vi "MF-101 Serial write and read on same channel.vi"() -> ()   [LabVIEW 8.6]
uses:
  <libdir>/resource/objmgr/ueidaq.rc
  vi.lib/UeiDaq/UeiDaqConfigureTimingForSimpleIO.vi
  vi.lib/UeiDaq/UeiDaqCreateSerialSession.vi
  vi.lib/UeiDaq/UeiDaqReadOneDigitalScanUInt16.vi
  vi.lib/UeiDaq/UeiDaqCreateDISession.vi
  vi.lib/UeiDaq/UeiDaqCreateDOSession.vi
  vi.lib/UeiDaq/UeiDaqWriteOneDigitalScanUInt16.vi
  vi.lib/UeiDaq/UeiDaqConfigureTimingForMessagingIO.vi
panel:
  out "DO raw data":u32[](array[numeric]) format="%b"
  out "Total scans":u32
  in  "TRIGOUT":bool
  out "DI TTL Port":bool[][](array[boolean])
  out "Total scans acquired":u32
  in  "Digital Output Resource":string
  in  "Digital Input Resource":string
  out "Available bytes":i32[](array[numeric])
  in  "Append":bool
  in  "Clear":bool
  out "Timeout":bool
  in  "Bits per second":i32(ring) items=["110 bitsPerSecond", "300 bitsPerSecond", "600 bitsPerSecond", "1200 bitsPerSecond", "2400 bitsPerSecond", "4800 bitsPerSecond", "9600 bitsPerSecond", "14400 bitsPerSecond", "19200 bits PerSecond", "28800 bitsPerSecond", "38400 bitsPerSecond", "57600 bitsPerSecond", "115200 bitsPerSecond", "128000 bitsPerSecond", "256000 bitsPerSecond"]
  in  "Stop bits":i32(ring) items=["1 stop bit", "1.5 stop bits", "2 stop bits"]
  in  "Parity":i32(ring) items=["None", "Odd", "Even"]
  in  "Data bits":i32(ring) items=["5 data bits", "6 data bits", "7 data bits", "8 data bits"]
  out "string from serial port":string
  in  "String to send to serial port":string
  in  "Send":bool
  out "return count":i32
  out "device name":string
  in  "Serial Resource":string
  in  "stop":bool
  # "MF-101 Write & Read Serial Port"
  # "1/ Set the resource name -->"
  # "TRUE  = RS232\nFALSE = RS422/485"
  # "2/ Configure Serial port -->"
  # "3/ Send/Receive -->"
  # "Device info"
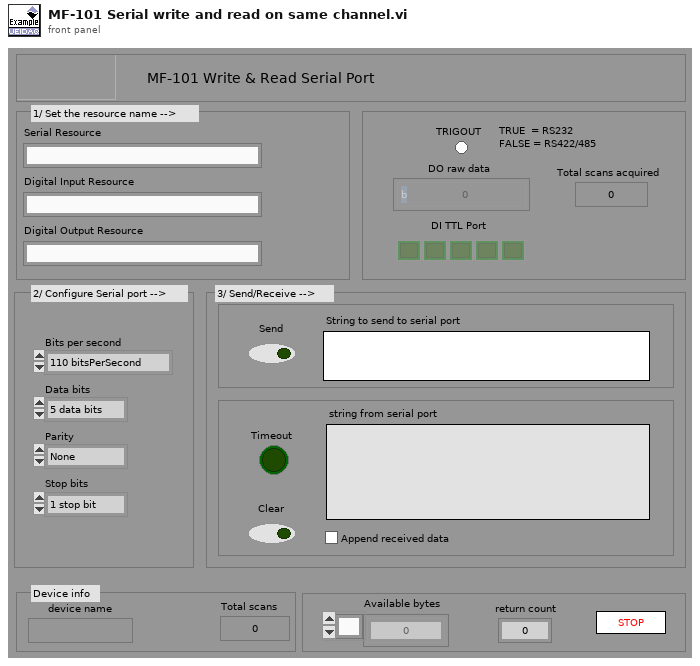
[diagram p1: front panel]
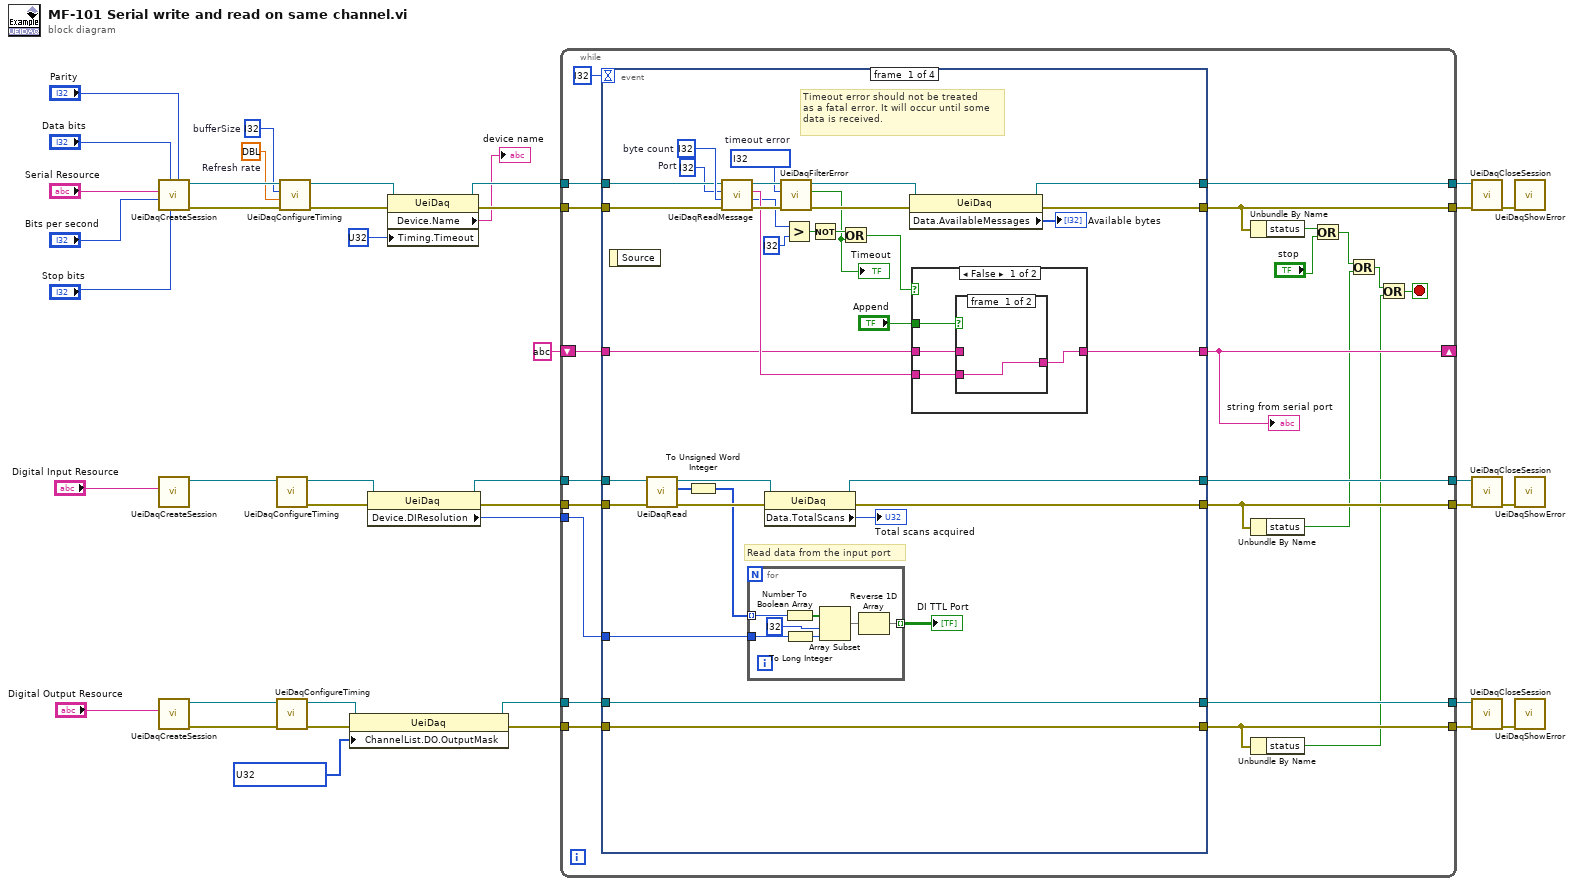
[diagram p0: block diagram]
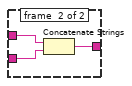
[diagram p2: hidden frame]
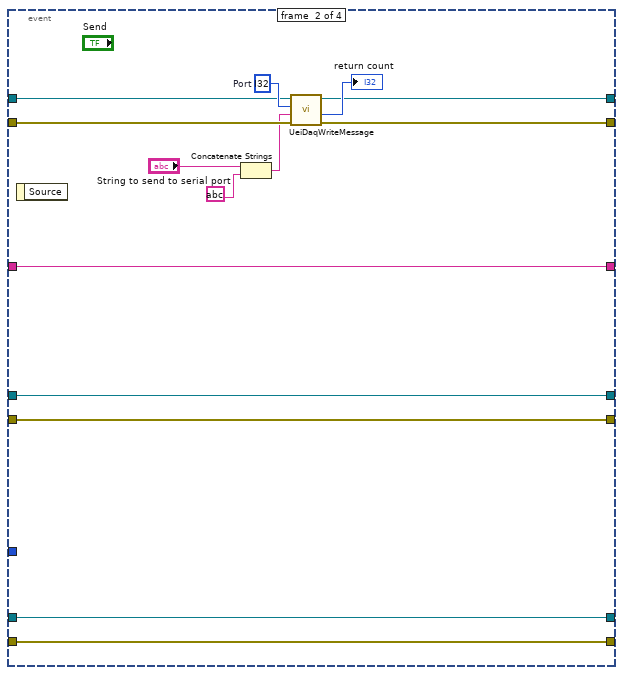
[diagram p4: hidden frame]
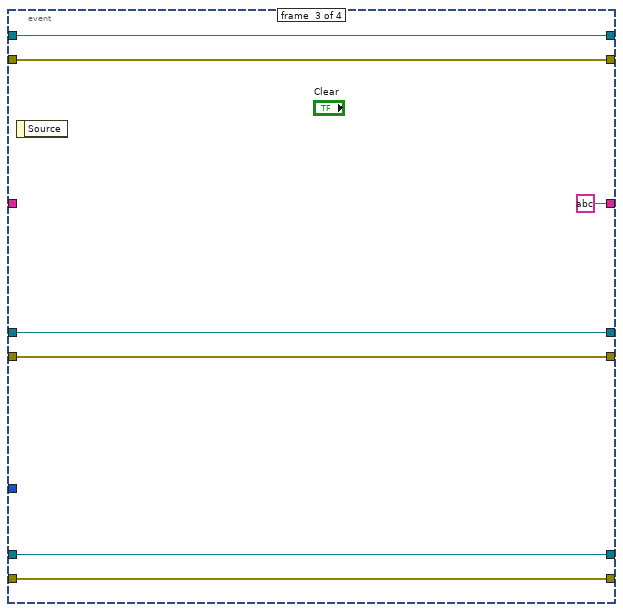
[diagram p5: hidden frame]
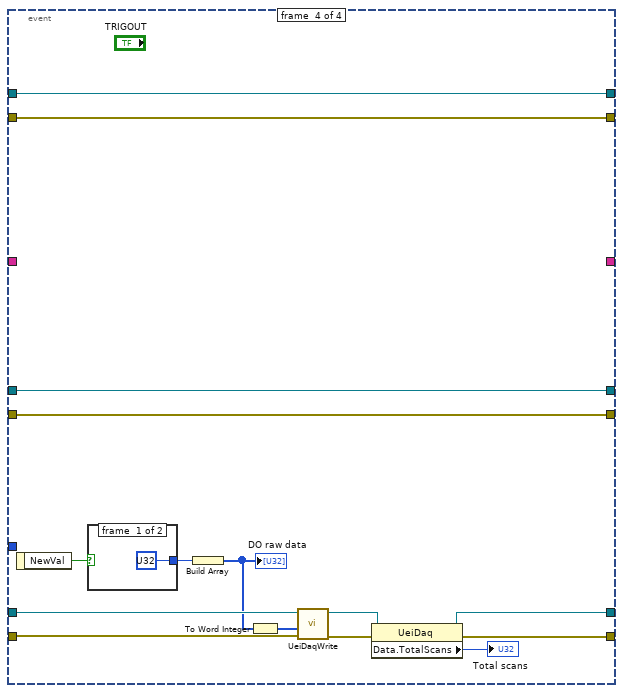
[diagram p6: hidden frame]
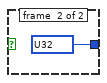
[diagram p7: hidden frame]
diagram:
  w1 = i32 ?  # bufferSize
  w2 = dbl ?  # Refresh rate
  n1 = call-poly "UeiDaqCreateSession.vi"("Parity"="Parity", "Stop bits"="Stop bits", "Data bits"="Data bits", "Bits per second"="Bits per second", "Resource"="Serial Resource") -> ("error out"=w37:errorcluster, "UeiDaq Refnum Out"=w38:refnum<k20>)  [unwired: 4 in, 1 out]
  n2 = call-poly "UeiDaqCreateSession.vi"("Resource"="Digital Input Resource") -> ("UeiDaq Refnum Out"=w8:refnum<k20>)  [unwired: 2 in, 8 out]
  n3 = call-poly "UeiDaqCreateSession.vi"("Resource"="Digital Output Resource") -> ("error out"=w22:errorcluster, "UeiDaq Refnum Out"=w23:refnum<k20>)  [unwired: 3 in, 6 out]
  n4 = call-poly "UeiDaqConfigureTiming.vi"("UeiDaq Refnum In"=w8) -> ("error out"=w6:errorcluster, "UeiDaq Refnum Out"=w7:refnum<k20>)  [unwired: 2 in, 7 out]
  n5 = call-poly "UeiDaqConfigureTiming.vi"("error in (no error)"=w22, "UeiDaq Refnum In"=w23) -> ("error out"=w20:errorcluster, "UeiDaq Refnum Out"=w21:refnum<k20>)  [unwired: 1 in, 7 out]
  n6 = call-poly "UeiDaqConfigureTiming.vi"("error in (no error)"=w37, "Refresh rate"=w2, "bufferSize"=w1, "UeiDaq Refnum In"=w38) -> ("error out"=w33:errorcluster, "UeiDaq Refnum Out"=w35:refnum<k20>)  [unwired: 6 out]
  n7 = property class="UeiDaq"(reference=w21, error in=w20, "ChannelList.DO.OutputMask"=u32[] ? ("Output Mask")) -> (reference out=w11:refnum<k20>, error out=w10:errorcluster)
  n8 = property class="UeiDaq"(reference=w7, error in=w6) -> (reference out=w3:refnum<k20>, error out=w4:errorcluster, "Device.DIResolution"=w5:u32)
  n9 = property class="UeiDaq"(reference=w35, error in=w33, "Timing.Timeout"=u32 ? ("Timing:Timeout")) -> (reference out=w34:refnum<k20>, error out=w32:errorcluster, "Device.Name"=→"device name":string)
  n10 = while {
    tunnel: w34 -> [w62]
    tunnel: w32 -> [w63]
    tunnel: [w59] -> w31
    tunnel: [w60] -> w30
    shift-right: [w56] -> _
    shift-left: string ? ("Message") -> [w57]
    tunnel: w3 -> [w55]
    tunnel: w4 -> [w54]
    tunnel: w11 -> [w50]
    tunnel: w10 -> [w49]
    tunnel: w5 -> [w53]
    tunnel: [w52] -> w16
    tunnel: [w51] -> w15
    tunnel: [w48] -> w13
    tunnel: [w47] -> w12
    stop <- w41 stop-if-true
    n11 = event shown="[3] \"TRIGOUT\": Value Change" {
      selector: _ -> [_ _ _ _]
      dyn-events: _ -> [_ _ _ _]
      timeout: i32 ? -> [_ _ _ _]
      tunnel: w63 -> [w96 w125 w129 w136]
      tunnel: w62 -> [w97 w126 w130 w137]
      tunnel: [w90 w123 _ w137] -> w60
      tunnel: [w88 w124 w129 w136] -> w59
      tunnel: [w86 w119 string ? ("Message") _] -> w56
      tunnel: w57 -> [w85 w119 _ _]
      tunnel: w55 -> [w75 w116 w134 w139]
      tunnel: w54 -> [w76 w115 w133 w138]
      tunnel: [w74 w116 w134 w139] -> w52
      tunnel: w53 -> [w73 _ _ _]
      tunnel: [w72 w115 w133 w138] -> w51
      tunnel: w50 -> [w71 w118 w132 w147]
      tunnel: w49 -> [w70 w117 w131 w146]
      tunnel: [w71 w118 w132 w145] -> w48
      tunnel: [w70 w117 w131 w144] -> w47
      tunnel: [_ _ w130 _] -> _
      event #0 {
        w83 = i32 ?  # Port
        w92 = i32 ?  # timeout error
        w98 = i32 ?  # byte count
        # "Read data from the input port"
        # "Timeout error should not be treated\nas a fatal error. It will occur until some\ndata is received."
        n12 = event-data() -> ()  [unwired: 2 out]
        n13 = call-poly "UeiDaqRead.vi"("error in (no error)"=w76, "UeiDaq Refnum In"=w75) -> ("error out"=w78:errorcluster, "Raw Data"=w81:i16[], "UeiDaq Refnum Out"=w79:refnum<k20>)  [unwired: 7 out]
        n14 = To Unsigned Word Integer(number=w81) -> (unsigned 16bit integer=w77:u16[])
        n15 = call "UeiDaqReadMessage.vi"("error in (no error)"=w96, "byte count"=w98, "Port"=w83, "UeiDaq Refnum In"=w97) -> ("error out"=w94:errorcluster, "return count"=w69:i32, "Message"=w93:string, "UeiDaq Refnum Out"=w95:refnum<k20>)  [unwired: 4 out]
        n16 = for {
          tunnel: w77 -> [w105] mode=indexing
          tunnel: w73 -> [w102]
          tunnel: [w100] -> w82 mode=indexing
          n17 = Number To Boolean Array(number=w105) -> (Boolean array=w104:bool[])
          n18 = To Long Integer(number=w102) -> (32bit integer=w99:i32)
          n19 = Array Subset(array=w104, index=i32 ?, length=w99) -> (w101:bool[])
          n20 = Reverse 1D Array(array=w101) -> (reversed array=w100:bool[])
        }
        "DI TTL Port" <- w82
        n21 = property class="UeiDaq"(reference=w79, error in=w78) -> (reference out=w74:refnum<k20>, error out=w72:errorcluster, "Data.TotalScans"=→"Total scans acquired":u32)
        n22 = call "UeiDaqFilterError.vi"("error in (no error)"=w94, "Error to filter"=w92, "UeiDaq Refnum In"=w95) -> ("error out"=w89:errorcluster, "Error filtered"=w65:bool, "UeiDaq Refnum Out"=w91:refnum<k20>)  [unwired: 6 out]
        "Timeout" <- w65
        n23 = Greater?(x=w69, y=i32 ?) -> (0:w67:bool)
        n24 = Not(x=w67) -> (.not. x?=w66:bool)
        n25 = Or(x=w66, y=w65) -> (x .or. y?=w64:bool)
        n26 = property class="UeiDaq"(reference=w91, error in=w89) -> (reference out=w90:refnum<k20>, error out=w88:errorcluster, "Data.AvailableMessages"=→"Available bytes":i32[])
        n27 = case shown="False" w64 {
          tunnel: w93 -> [w108 _]
          tunnel: "Append" -> [w109 _]
          tunnel: [w107 w114] -> w86
          tunnel: w85 -> [w106 w114]
          frame #0 {
            n28 = case shown="True" w109 {
              tunnel: w108 -> [w110 w113]
              tunnel: [w110 w112] -> w107
              tunnel: w106 -> [_ w111]
              frame #0 {
              }
              frame #1 {
                n29 = Concatenate Strings(w111, w113) -> (w112:string)
              }
            }
          }
          frame #1 {
          }
        }
      }
      event #1 {
        w128 = i32 ?  # Port
        n30 = event-data() -> ()  [unwired: 2 out]
        n31 = Concatenate Strings("String to send to serial port", string ?) -> (w120:string)
        n32 = call "UeiDaqWriteMessage.vi"("error in (no error)"=w125, "Message"=w120, "Port"=w128, "UeiDaq Refnum In"=w126) -> ("error out"=w124:errorcluster, "return count"=→"return count":i32, "UeiDaq Refnum Out"=w123:refnum<k20>)  [unwired: 5 out]
      }
      event #2 {
        n33 = event-data() -> ()  [unwired: 2 out]
      }
      event #3 {
        n34 = event-data() -> ("NewVal"=w140:bool)  [unwired: 1 out]
        n35 = case shown="True" w140 {
          tunnel: [u32 ? u32 ?] -> w143
          frame #0 {
          }
          frame #1 {
          }
        }
        n36 = Build Array(w143) -> (w141:u32[])
        "DO raw data" <- w141
        n37 = To Word Integer(number=w141) -> (16bit integer=w142:i16[])
        n38 = call-poly "UeiDaqWrite.vi"("error in (no error)"=w146, "Digital Data"=w142, "UeiDaq Refnum In"=w147) -> ("error out"=w149:errorcluster, "UeiDaq Refnum Out"=w150:refnum<k20>)  [unwired: 7 out]
        n39 = property class="UeiDaq"(reference=w150, error in=w149) -> (reference out=w145:refnum<k20>, error out=w144:errorcluster, "Data.TotalScans"=→"Total scans":u32)
      }
    }
    "string from serial port" <- w56
    n40 = Unbundle By Name(w59) -> ("status"=w61:bool)
    n41 = Unbundle By Name(w51) -> ("status"=w44:bool)
    n42 = Unbundle By Name(w47) -> ("status"=w42:bool)
    n43 = Or(x=w61, y="stop") -> (x .or. y?=w45:bool)
    n44 = Or(x=w45, y=w44) -> (x .or. y?=w43:bool)
    n45 = Or(x=w43, y=w42) -> (x .or. y?=w41:bool)
  }
  n46 = call "UeiDaqCloseSession.vi"("error in (no error)"=w31, "UeiDaq Refnum In"=w30) -> ("error out"=w39:errorcluster)  [unwired: 1 in, 8 out]
  n47 = call "UeiDaqCloseSession.vi"("error in (no error)"=w15, "UeiDaq Refnum In"=w16) -> ("error out"=w17:errorcluster)  [unwired: 1 in, 8 out]
  n48 = call "UeiDaqCloseSession.vi"("error in (no error)"=w12, "UeiDaq Refnum In"=w13) -> ("error out"=w14:errorcluster)  [unwired: 1 in, 8 out]
  n49 = call "UeiDaqShowError.vi"("error in (no error)"=w39) -> ()  [unwired: 2 in, 9 out]
  n50 = call "UeiDaqShowError.vi"("error in (no error)"=w17) -> ()  [unwired: 2 in, 9 out]
  n51 = call "UeiDaqShowError.vi"("error in (no error)"=w14) -> ()  [unwired: 2 in, 9 out]
